vi "System Commands.vi"() -> ()   [LabVIEW 2013]
uses:
  <vilib>/LabVIEW Hacker/LINX/Private/Device/Device.lvlib
panel:
  in  "IP Address":string="192.168.1.27"
  in  "Port":u16
  out "Error Out":errorcluster
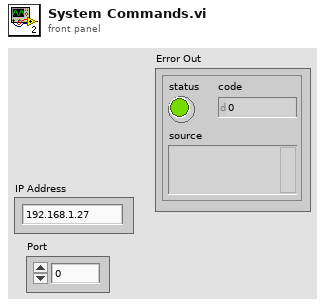
[diagram p1: front panel]
types:
  T1 = typedef "LVH-LINX.lvlib/Device.lvlib/LINX Device Config.ctl" = cluster{"Interface":T2, "COM Port":refnum<visa-resource-name>, "TCP Configuration":T3, "Device Family":T4, "Device ID":u8, "Device Name":string, "TCP Ref":refnum<k5>}
  T2 = typedef "LVH-LINX.lvlib/Interface.ctl" = enum16{"Serial", "TCP"}
  T3 = typedef "LVH-LINX.lvlib/Device.lvlib/TCP Config.ctl" = cluster{"IP Address":string, "Port":u16}
  T4 = typedef "LVH-LINX.lvlib/Device Family.ctl" = enum8{"National Instruments", "Digilent", "Arduino"}
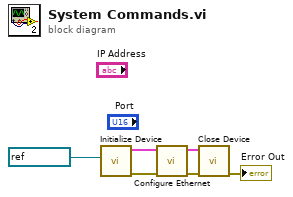
[diagram p0: block diagram]
diagram:
  n1 = call <vilib>:"Initialize Device.vi"("COM Port"=refnum<visa-resource-name> "COM6") -> ("Error Out"=w1:errorcluster, "LINX Device Config"=w4:T1)  [unwired: 8 in, 1 out]
  n2 = call <vilib>:"Configure Ethernet.vi"("Error In"=w1, "LINX Device Config"=w4) -> ("Error Out"=w2:errorcluster, "LINX Device Config"=w3:T1)  [unwired: 8 in]
  n3 = call <vilib>:"Close Device.vi"("Error In"=w2, "LINX Device Config"=w3) -> ("Error Out"=→"Error Out":errorcluster)  [unwired: 8 in, 1 out]
